vi "Ms to Time.vi"(1 "ms":i64) -> (0 "Time":string)   [LabVIEW 2016]
doc: "This VI takes the time in miliseconds and reformats it like a standard digital clock. This was used for autonomous logs so it can only show time in M:S:MS\n\nCreated by Team 4130 for use in the 2016-2017 FRC season"
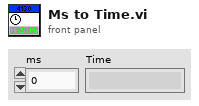
[diagram p1: front panel]
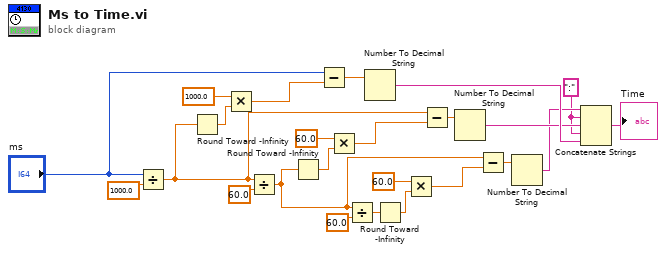
[diagram p0: block diagram]
diagram:
  w1 = ":" ("string")
  n1 = Divide(x="ms", y=1000.0) -> (x/y=w13:dbl)
  n2 = Round Toward -Infinity(1:w13) -> (0:w19:dbl)
  n3 = Multiply(x=1000.0, y=w19) -> (x*y=w17:dbl)
  n4 = Divide(x=w13, y=60.0) -> (x/y=w9:dbl)
  n5 = Round Toward -Infinity(1:w9) -> (0:w15:dbl)
  n6 = Subtract(x="ms", y=w17) -> (x-y=w8:dbl)
  n7 = Multiply(x=60.0, y=w15) -> (x*y=w14:dbl)
  n8 = Divide(x=w9, y=60.0) -> (x/y=w21:dbl)
  n9 = Number To Decimal String(number=w8) -> (decimal integer string=w4:string)  [unwired: 1 in]
  n10 = Round Toward -Infinity(1:w21) -> (0:w10:dbl)
  n11 = Multiply(x=60.0, y=w10) -> (x*y=w12:dbl)
  n12 = Subtract(x=w13, y=w14) -> (x-y=w7:dbl)
  n13 = Number To Decimal String(number=w7) -> (decimal integer string=w3:string)  [unwired: 1 in]
  n14 = Subtract(x=w9, y=w12) -> (x-y=w6:dbl)
  n15 = Number To Decimal String(number=w6) -> (decimal integer string=w2:string)  [unwired: 1 in]
  n16 = Concatenate Strings(w2, w1, w3, w1, w4) -> (→"Time":string)
